vi "execute.vi"(8 "error in (no error)":errorcluster, 9 "trajectory resonance in":refnum<class "GenericComponent.lvclass">, 10 "imaging mode in":refnum<class "GenericComponent.lvclass">, 11 "AdapterAK101022ImagingModeToTrajectory in":refnum<class "AdapterAK101022ImagingModeToTrajectory.lvclass">) -> (0 "error out":errorcluster, 1 "trajectory resonance out":refnum<class "GenericComponent.lvclass">, 2 "imaging mode out":refnum<class "GenericComponent.lvclass">, 3 "AdapterAK101022ImagingModeToTrajectory out":refnum<class "AdapterAK101022ImagingModeToTrajectory.lvclass">)   [LabVIEW 2010, in "AdapterAK101022ImagingModeToTrajectory.lvclass"]
uses:
  AdapterAK101022ImagingModeToTrajectory.lvclass
  common/classes/GenericComponent/GenericComponent/GenericComponent.lvclass
  ImagingMode/ImagingModeDL090130Frame/ImagingModeDL090130Frame/ImagingModeDL090130Frame.lvclass
  Trajectory/TrajectoryAK101022Resonance/TrajectoryAK101022Resonance/TrajectoryAK101022Resonance.lvclass
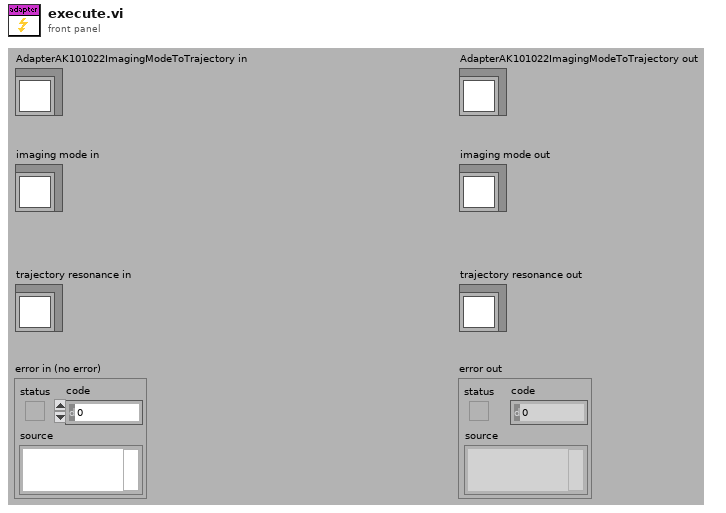
[diagram p1: front panel]
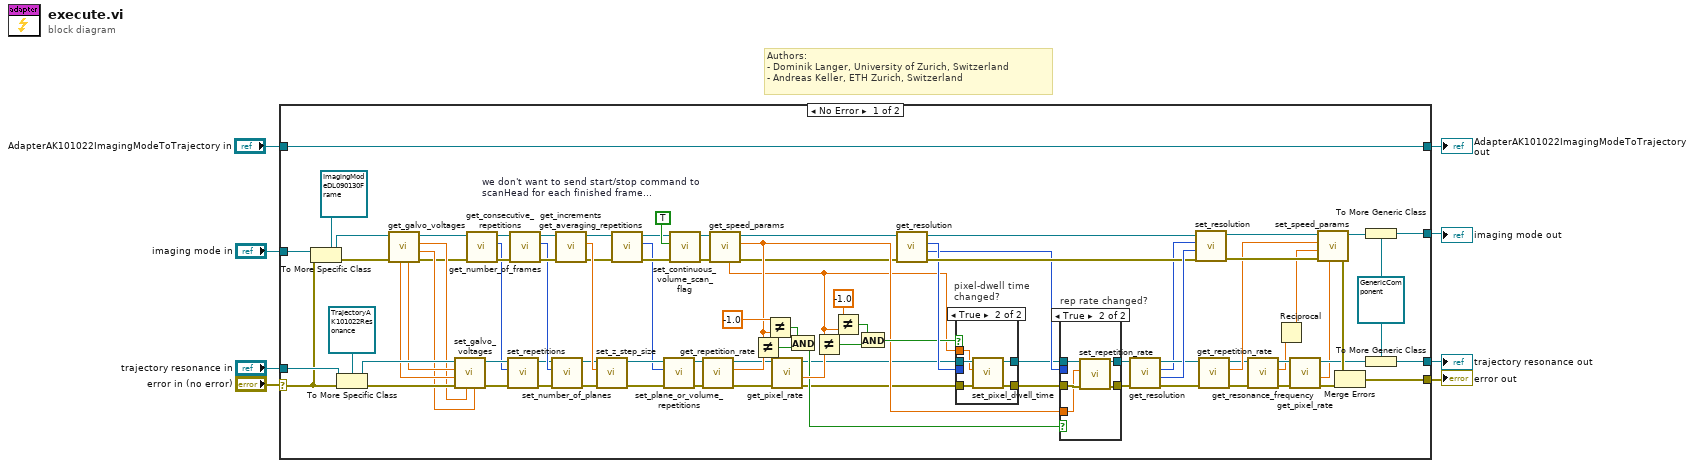
[diagram p0: block diagram]
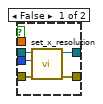
[diagram p2: hidden frame]
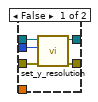
[diagram p3: hidden frame]
diagram:
  # "Authors: \n- Dominik Langer, University of Zurich, Switzerland\n- Andreas Keller, ETH Zurich, Switzerland"
  n1 = case shown="No Error" "error in (no error)" {
    selector: "error in (no error)" -> [w89 w118]
    tunnel: "AdapterAK101022ImagingModeToTrajectory in" -> [w97 w121]
    tunnel: [w97 w121] -> w6
    tunnel: [w91 w120] -> w4
    tunnel: "imaging mode in" -> [w94 w120]
    tunnel: [w92 w119] -> w2
    tunnel: "trajectory resonance in" -> [w96 w119]
    tunnel: [w81 w118] -> w1
    frame No Error {
      w38 = TRUE  # we don't want to send start/stop command to scanHead for each finished frame...
      w90 = refnum<class "GenericComponent.lvclass"> refnum ("GenericComponent.lvclass")
      n2 = To More Specific Class(target class=refnum<class "ImagingModeDL090130Frame.lvclass"> refnum ("DL090130FrameScanMode.lvclass"), reference=w94, error in=w89) -> (specific class reference=w23:refnum<class "ImagingModeDL090130Frame.lvclass">, error out=w22:errorcluster)
      n3 = To More Specific Class(target class=refnum<class "TrajectoryAK101022Resonance.lvclass"> refnum ("TrajectoryAK101022Resonance.lvclass"), reference=w96, error in=w89) -> (specific class reference=w21:refnum<class "TrajectoryAK101022Resonance.lvclass">, error out=w18:errorcluster)
      n4 = call-dynamic "get_galvo_voltages.vi"("error in (no error)"=w22, "ImagingModeDL090130Frame in"=w23) -> ("error out"=w12:errorcluster, "deltaVy(V)"=w14:dbl, "Vy0(V)"=w15:dbl, "ImagingModeDL090130Frame out"=w13:refnum<class "ImagingModeDL090130Frame.lvclass">, "Vz0(V)"=w17:dbl, "deltaVz(V)"=w16:dbl)  [unwired: 4 in]
      n5 = call-dynamic "set_galvo_voltages.vi"("deltaVy0(V)"=w14, "Vy0(V)"=w15, "error in (no error)"=w18, "deltaVz(V)"=w16, "Vz0(V)"=w17, "TrajectoryAK101022Resonance in"=w21) -> ("error out"=w19:errorcluster, "TrajectoryAK101022Resonance out"=w20:refnum<class "TrajectoryAK101022Resonance.lvclass">)  [unwired: 4 in]
      n6 = call-dynamic "get_consecutive_repetitions.vi"("error in (no error)"=w12, "ImagingModeDL090130Frame in"=w13) -> ("error out"=w10:errorcluster, "number of consecutive repetitions"=w9:i32, "ImagingModeDL090130Frame out"=w11:refnum<class "ImagingModeDL090130Frame.lvclass">)  [unwired: 7 in]
      n7 = call-dynamic "set_repetitions.vi"("error in (no error)"=w19, "repetitions"=w9, "GenericTrajectory in"=w20) -> ("error out"=w37:errorcluster, "GenericTrajectory out"=w36:refnum<class "TrajectoryAK101022Resonance.lvclass">)  [unwired: 7 in]
      n8 = call-dynamic "get_number_of_frames.vi"("error in (no error)"=w10, "ImagingModeDL090130Frame in"=w11) -> ("error out"=w44:errorcluster, "number of frames"=w42:i32, "ImagingModeDL090130Frame out"=w43:refnum<class "ImagingModeDL090130Frame.lvclass">)  [unwired: 7 in]
      n9 = call-dynamic "set_number_of_planes.vi"("error in (no error)"=w37, "Number of planes"=w42, "TrajectoryAK101022Resonance in"=w36) -> ("error out"=w34:errorcluster, "TrajectoryAK101022Resonance out"=w35:refnum<class "TrajectoryAK101022Resonance.lvclass">)  [unwired: 7 in]
      n10 = call-dynamic "get_increments.vi"("error in (no error)"=w44, "ImagingModeDL090130Frame in"=w43) -> ("error out"=w32:errorcluster, "step size"=w41:dbl[unit], "ImagingModeDL090130Frame out"=w31:refnum<class "ImagingModeDL090130Frame.lvclass">)  [unwired: 7 in]
      n11 = call-dynamic "set_z_step_size.vi"("error in (no error)"=w34, "z step size"=w41, "TrajectoryAK101022Resonance in"=w35) -> ("error out"=w28:errorcluster, "TrajectoryAK101022Resonance out"=w27:refnum<class "TrajectoryAK101022Resonance.lvclass">)  [unwired: 7 in]
      n12 = call-dynamic "get_averaging_repetitions.vi"("error in (no error)"=w32, "ImagingModeDL090130Frame in"=w31) -> ("error out"=w29:errorcluster, "averaging repetitions"=w24:i32, "ImagingModeDL090130Frame out"=w30:refnum<class "ImagingModeDL090130Frame.lvclass">)  [unwired: 7 in]
      n13 = call-dynamic "set_plane_or_volume_repetitions.vi"("error in (no error)"=w28, "repetitions per frame"=w24, "TrajectoryAK101022Resonance in"=w27) -> ("error out"=w26:errorcluster, "TrajectoryAK101022Resonance out"=w25:refnum<class "TrajectoryAK101022Resonance.lvclass">)  [unwired: 7 in]
      n14 = call "set_continuous_volume_scan_flag.vi"("error in (no error)"=w29, "perform continuous volume scan?"=w38, "ImagingModeDL090130Frame in"=w30) -> ("error out"=w40:errorcluster, "ImagingModeDL090130Frame out"=w39:refnum<class "ImagingModeDL090130Frame.lvclass">)  [unwired: 7 in]
      n15 = call-dynamic "get_repetition_rate.vi"("error in (no error)"=w26, "GenericTrajectory in"=w25) -> ("error out"=w62:errorcluster, "repetition rate"=w78:dbl[unit], "GenericTrajectory out"=w63:refnum<class "TrajectoryAK101022Resonance.lvclass">)  [unwired: 7 in]
      n16 = call-dynamic "get_speed_params.vi"("error in (no error)"=w40, "ImagingModeDL090130Frame in"=w39) -> ("error out"=w48:errorcluster, "frame rate"=w49:dbl[unit], "ImagingModeDL090130Frame out"=w47:refnum<class "ImagingModeDL090130Frame.lvclass">, "pixel dwell time"=w33:dbl[unit])  [unwired: 4 in, 2 out]
      n17 = Not Equal?(x=w49, y=w78) -> (x != y?=w57:bool)
      n18 = Not Equal?(x=dbl[unit] -1.0, y=w49) -> (x != y?=w56:bool)
      n19 = call-dynamic "get_pixel_rate.vi"("error in (no error)"=w62, "TrajectoryAK101022Resonance in"=w63) -> ("error out"=w46:errorcluster, "pixel dwell time"=w61:dbl[unit], "TrajectoryAK101022Resonance out"=w45:refnum<class "TrajectoryAK101022Resonance.lvclass">)  [unwired: 6 in, 1 out]
      n20 = And(x=w56, y=w57) -> (x .and. y?=w50:bool)
      n21 = Not Equal?(x=w33, y=w61) -> (x != y?=w54:bool)
      n22 = Not Equal?(x=dbl[unit] -1.0, y=w33) -> (x != y?=w53:bool)
      n23 = And(x=w53, y=w54) -> (x .and. y?=w52:bool)
      n24 = call-dynamic "get_resolution.vi"("error in (no error)"=w48, "ImagingModeDL090130Frame in"=w47) -> ("error out"=w87:errorcluster, "y resolution"=w84:i32, "x resolution"=w86:i32, "ImagingModeDL090130Frame out"=w85:refnum<class "ImagingModeDL090130Frame.lvclass">)  [unwired: 6 in]
      n25 = case "pixel-dwell time changed?" shown="True" w52 {
        tunnel: w86 -> [w102 _]
        tunnel: w45 -> [w101 w104]
        tunnel: w46 -> [w100 w107]
        tunnel: [w99 w106] -> w59
        tunnel: [w98 w105] -> w58
        tunnel: w33 -> [_ w103]
        frame False {
          n26 = call-dynamic "set_x_resolution.vi"("error in (no error)"=w100, "x resolution"=w102, "TrajectoryAK101022Resonance in"=w101) -> ("error out"=w99:errorcluster, "TrajectoryAK101022Resonance out"=w98:refnum<class "TrajectoryAK101022Resonance.lvclass">)  [unwired: 7 in]
        }
        frame True {
          n27 = call-dynamic "set_pixel_dwell_time.vi"("error in (no error)"=w107, "pixel-dwell time"=w103, "TrajectoryAK101022Resonance in"=w104) -> ("error out"=w106:errorcluster, "TrajectoryAK101022Resonance out"=w105:refnum<class "TrajectoryAK101022Resonance.lvclass">)  [unwired: 7 in]
        }
      }
      n28 = case "rep rate changed?" shown="True" w50 {
        tunnel: w59 -> [w112 w115]
        tunnel: w58 -> [w111 w116]
        tunnel: w84 -> [w110 _]
        tunnel: [w109 w114] -> w80
        tunnel: [w108 w117] -> w79
        tunnel: w49 -> [_ w113]
        frame False {
          n29 = call-dynamic "set_y_resolution.vi"("error in (no error)"=w112, "y resolution"=w110, "TrajectoryAK101022Resonance in"=w111) -> ("error out"=w109:errorcluster, "TrajectoryAK101022Resonance out"=w108:refnum<class "TrajectoryAK101022Resonance.lvclass">)  [unwired: 7 in]
        }
        frame True {
          n30 = call-dynamic "set_repetition_rate.vi"("error in (no error)"=w115, "repetition rate"=w113, "TrajectoryAK101022Resonance in"=w116) -> ("error out"=w114:errorcluster, "TrajectoryAK101022Resonance out"=w117:refnum<class "TrajectoryAK101022Resonance.lvclass">)  [unwired: 7 in]
        }
      }
      n31 = call-dynamic "get_resolution.vi"("error in (no error)"=w80, "TrajectoryAK101022Resonance in"=w79) -> ("error out"=w83:errorcluster, "y resolution"=w88:i32, "x resolution"=w60:i32, "TrajectoryAK101022Resonance out"=w82:refnum<class "TrajectoryAK101022Resonance.lvclass">)  [unwired: 6 in]
      n32 = call-dynamic "set_resolution.vi"("error in (no error)"=w87, "y"=w88, "x"=w60, "ImagingModeDL090130Frame in"=w85) -> ("error out"=w77:errorcluster, "ImagingModeDL090130Frame out"=w75:refnum<class "ImagingModeDL090130Frame.lvclass">)  [unwired: 6 in]
      n33 = call-dynamic "get_repetition_rate.vi"("error in (no error)"=w83, "GenericTrajectory in"=w82) -> ("error out"=w69:errorcluster, "repetition rate"=w76:dbl[unit], "GenericTrajectory out"=w67:refnum<class "TrajectoryAK101022Resonance.lvclass">)  [unwired: 7 in]
      n34 = call-dynamic "get_resonance_frequency.vi"("error in (no error)"=w69, "TrajectoryAK101022Resonance in"=w67) -> ("error out"=w68:errorcluster, "resonance frequency"=w65:dbl[unit], "TrajectoryAK101022Resonance out"=w66:refnum<class "TrajectoryAK101022Resonance.lvclass">)  [unwired: 7 in]
      n35 = Reciprocal(x=w65) -> (1/x=w64:dbl[unit])
      n36 = call-dynamic "get_pixel_rate.vi"("error in (no error)"=w68, "TrajectoryAK101022Resonance in"=w66) -> ("error out"=w72:errorcluster, "pixel dwell time"=w70:dbl[unit], "TrajectoryAK101022Resonance out"=w71:refnum<class "TrajectoryAK101022Resonance.lvclass">)  [unwired: 6 in, 1 out]
      n37 = call-dynamic "set_speed_params.vi"("pixel-dwell time"=w70, "error in (no error)"=w77, "line-scan time"=w64, "frame rate"=w76, "ImagingModeDL090130Frame in"=w75) -> ("error out"=w73:errorcluster, "ImagingModeDL090130Frame out"=w74:refnum<class "ImagingModeDL090130Frame.lvclass">)  [unwired: 5 in]
      n38 = Merge Errors(w73, w72) -> (w81:errorcluster)
      n39 = To More Generic Class(target class=w90, reference=w74) -> (generic class reference=w91:refnum<class "GenericComponent.lvclass">)
      n40 = To More Generic Class(target class=w90, reference=w71) -> (generic class reference=w92:refnum<class "GenericComponent.lvclass">)
    }
    frame Error {
    }
  }
  "error out" <- w1
  "AdapterAK101022ImagingModeToTrajectory out" <- w6
  "imaging mode out" <- w4
  "trajectory resonance out" <- w2
